vi "Query Arb Waveform Capabilities 64 [ARB64].vi"(8 "error in (no error)":errorcluster, 11 "CS++Fgen in":refnum<class "CS++Fgen.lvclass">) -> (0 "error out":errorcluster, 1 "waveform quantum":i32, 2 "max number of waveforms":i32, 3 "CS++Fgen out":refnum<class "CS++Fgen.lvclass">, 4 "max waveform size":i64, 6 "min waveform size":i64)   [LabVIEW 2013, in "CS++Fgen.lvlib" / "CS++Fgen.lvclass"]
doc: "This VI returns the properties of the function generator that are related to creating arbitrary waveforms. These properties are the maximum number of waveforms, waveform quantum, minimum waveform size, and maximum waveform size.\n\nThis VI is a 64-bit version of IviFgen Query Arb Waveform Capabilities [ARB] VI.\n\nNote:\n\n(1) This VI is part of the IviFgenArbWfmSize64 [ARB64] extension group."
uses:
  CS++Fgen.lvclass
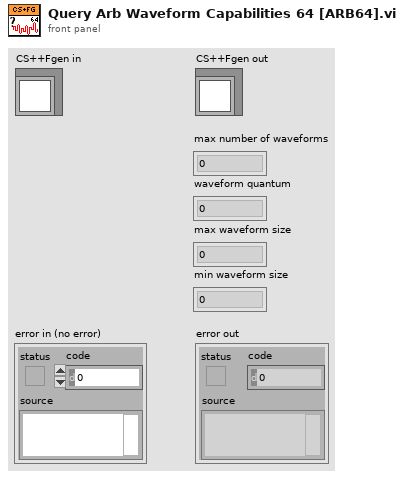
[diagram p1: front panel]
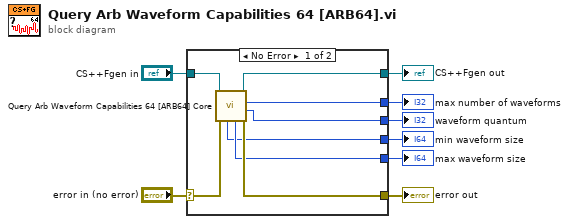
[diagram p0: block diagram]
diagram:
  n1 = case shown="No Error" "error in (no error)" {
    selector: "error in (no error)" -> [w14 w18]
    tunnel: [w13 w18] -> w7
    tunnel: [w15 w17] -> w5
    tunnel: "CS++Fgen in" -> [w16 w17]
    tunnel: [w11 _] -> w4
    tunnel: [w12 _] -> w3
    tunnel: [w9 _] -> w2
    tunnel: [w10 _] -> w1
    frame No Error {
      n2 = call-dynamic "Query Arb Waveform Capabilities 64 [ARB64] Core.vi"("error in (no error)"=w14, "CS++Fgen in"=w16) -> ("error out"=w13:errorcluster, "waveform quantum"=w9:i32, "max number of waveforms"=w12:i32, "CS++Fgen out"=w15:refnum<class "CS++Fgen.lvclass">, "max waveform size"=w11:i64, "min waveform size"=w10:i64)  [unwired: 4 in]
    }
    frame Error {
    }
  }
  "error out" <- w7
  "CS++Fgen out" <- w5
  "max number of waveforms" <- w3
  "waveform quantum" <- w2
  "max waveform size" <- w4
  "min waveform size" <- w1
